vi "dvp Vi Get Rgb Gain State.vi"(10 "pState":i32, 11 "handle":u32) -> (2 "pState out":i32, 3 "function return":u32(ring))   [LabVIEW 2018, in "LabViewDVPCamera.lvlib"]
doc: "LabviewDvp2Api dvpStatus dvpViGetRgbGainState(dvpHandle handle, BOOL *pState);"
uses:
  LabViewDVPCamera.lvlib
  LabViewDVPCamera/LabViewDVPCamera.dll
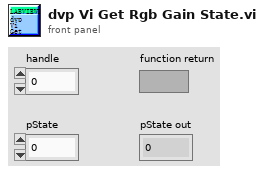
[diagram p1: front panel]
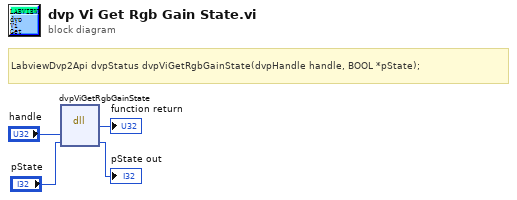
[diagram p0: block diagram]
diagram:
  # "LabviewDvp2Api dvpStatus dvpViGetRgbGainState(dvpHandle handle, BOOL *pState);"
  n1 = dll-call lib="C:/Program Files (x86)/DVP2 Labview cn 64/Sample/LabViewDVPCamera/LabViewDVPCamera.*" fn="dvpViGetRgbGainState"("handle"="handle", "pState"="pState") -> (→"function return":u32, "pState"=→"pState out":i32)  [unwired: 4 in, 2 out]
